vi "box detection.vi"(0 "PWM Ref In 2":T1, 1 "Angle":dbl, 2 "Distance":dbl, 3 "error in (no error) 2":errorcluster) -> (10 "error out 2":errorcluster)   [LabVIEW 2014]
uses:
  <vilib>/myRIO/Instrument Drivers/Onboard IO/PWM/typedefs/PWM Reference.ctl
  <vilib>/myRIO/Common/Instrument Driver Framework/Utilities/typedefs/myRIO Generic Hardware Reference.ctl
  <vilib>/myRIO/Common/Instrument Driver Framework/Utilities/typedefs/Hardware Version Enum.ctl
  <vilib>/myRIO/Common/Instrument Driver Framework/Utilities/typedefs/myRIO v1.0 Reference.ctl
  <vilib>/myRIO/Common/Instrument Driver Framework/Utilities/typedefs/Generic FPGA Reference.ctl
  <vilib>/myRIO/Common/Instrument Driver Framework/myRIO v1.0/PWM/typedefs/PWM Channels Enum.ctl
  <vilib>/myRIO/Instrument Drivers/Onboard IO/PWM/typedefs/PWM Configuration.ctl
  <vilib>/myRIO/Instrument Drivers/Onboard IO/AI/typedefs/AI Reference.ctl
  <vilib>/myRIO/Common/Instrument Driver Framework/myRIO v1.0/AI/typedefs/AI Channels List.ctl
  <vilib>/myRIO/Common/Instrument Driver Framework/myRIO v1.0/AI/typedefs/AI Channels Enum.ctl
  <vilib>/myRIO/Common/Instrument Driver Framework/Utilities/typedefs/Analog Scaling Constants List.ctl
  <vilib>/myRIO/Common/Instrument Driver Framework/Utilities/typedefs/Analog Scaling Constants.ctl
  <vilib>/userdefined/High Color/nirio_resource_hc.ctl
  <vilib>/myRIO/Common/Instrument Driver Framework/Utilities/vis/Is FPGA Ref Available.vi
  <vilib>/myRIO/Common/Instrument Driver Framework/myRIO v1.0/AI/vis/myRIO v1.1 Open AI.vi
  <vilib>/myRIO/Instrument Drivers/Onboard IO/AI/vis/Read.vi
  <vilib>/myRIO/Common/Instrument Driver Framework/Utilities/vis/Validate Channels.vi
  <vilib>/myRIO/Common/Instrument Driver Framework/myRIO v1.0/AI/vis/myRIO v1.0 Reserve AI.vi
  <vilib>/myRIO/Common/Instrument Driver Framework/myRIO v1.0/AI/vis/myRIO v1.0 Build MUX Configuration AI.vi
  <vilib>/myRIO/Common/Instrument Driver Framework/myRIO v1.0/Resource Manager/vis/myRIO v1.0 Reserve Channel List.vi
  <vilib>/myRIO/Common/Instrument Driver Framework/myRIO v1.0/Resource Manager/vis/myRIO v1.0 Reserve Channel.vi
  <vilib>/myRIO/Common/Instrument Driver Framework/myRIO v1.0/Resource Manager/vis/myRIO v1.0 Unreserve Channel.vi
  <vilib>/myRIO/Common/Instrument Driver Framework/myRIO v1.0/Resource Manager/vis/myRIO v1.0 Build Mutex Name.vi
  <vilib>/Utility/VariantDataType/GetNumericInfo.vi
  <vilib>/Utility/error.llb/Error Cluster From Error Code.vi
  <vilib>/myRIO/Common/Instrument Driver Framework/myRIO v1.0/myRIO v1.1 Open.vi
  <vilib>/myRIO/Common/Instrument Driver Framework/myRIO v1.0/AI/vis/myRIO v1.0 Get Scaling Constants AI.vi
  <vilib>/myRIO/Common/Instrument Driver Framework/Utilities/vis/IO Manager.vi
  <vilib>/myRIO/Common/Instrument Driver Framework/Utilities/vis/Configuration Manager.vi
  <vilib>/myRIO/Common/Instrument Driver Framework/myRIO v1.0/myRIO v1.0 Close.vi
  <vilib>/myRIO/Common/Instrument Driver Framework/myRIO v1.0/AI/vis/myRIO v1.0 Read AI.vi
  <vilib>/myRIO/Express VI/Onboard IO/AI/AI Express VI.xnode
  <vilib>/myRIO/Instrument Drivers/Onboard IO/AI/vis/myRIO AI Open.xnode
  <vilib>/ptbypt/NI_PtbyPt.lvlib
  <vilib>/myRIO/Instrument Drivers/Onboard IO/AI/AI.lvlib
  <vilib>/myRIO/Instrument Drivers/Onboard IO/PWM/PWM.lvlib
panel:
  out "color":string
  in  "Min range":dbl
  in  "Box is found":bool
  out "range":dbl format="%_3g"
  in  "Koffset [cm]":dbl
  in  "Kscale [cm-V]":dbl=27.5
  out "Vo [V]":dbl format="%.2f"
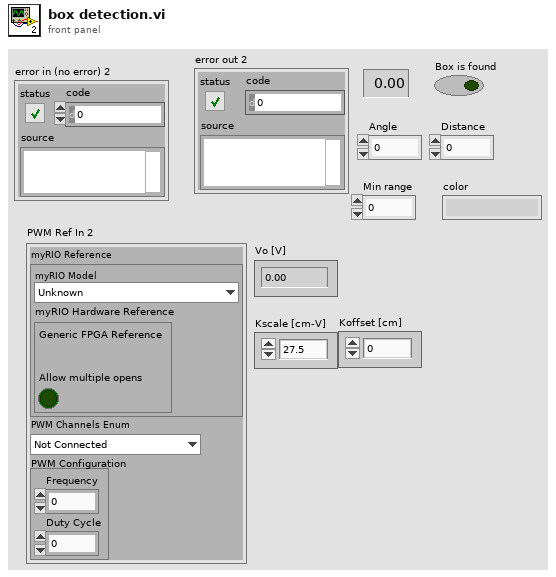
[diagram p1: front panel]
types:
  T1 = typedef "PWM.lvlib/PWM Reference.ctl" = cluster{"myRIO Reference":T2, "PWM Channels Enum":T6, "PWM Configuration":T7}
  T2 = typedef "myRIO Generic Hardware Reference.ctl" = cluster{"myRIO Model":T3, "myRIO Hardware Reference":T4}
  T3 = typedef "Hardware Version Enum.ctl" = enum16{"Unknown", "myRIO-1900", "myRIO-1950"}
  T4 = typedef "myRIO v1.0 Reference.ctl" = cluster{"Generic FPGA Reference":T5, "Allow multiple opens":bool}
  T5 = typedef "Generic FPGA Reference.ctl" = refnum<k20>
  T6 = typedef "PWM Channels Enum.ctl" = enum16{"Not Connected", "C/PWM0", "C/PWM1", "A/PWM0", "A/PWM1", "A/PWM2", "B/PWM0", "B/PWM1", "B/PWM2"}
  T7 = typedef "PWM.lvlib/PWM Configuration.ctl" = cluster{"Frequency":dbl, "Duty Cycle":dbl}
  T8 = typedef "AI.lvlib/AI Reference.ctl" = cluster{"myRIO Reference":T2, "AI Channels List":T9, "AI Scaling Constants List":T11}
  T9 = typedef "AI Channels List.ctl" = T10[]
  T10 = typedef "AI Channels Enum.ctl" = enum16{"Not Connected", "AudioIn/Left", "AudioIn/Right", "C/AI0", "C/AI1", "A/AI0", "A/AI1", "A/AI2", "A/AI3", "B/AI0", "B/AI1", "B/AI2", "B/AI3"}
  T11 = typedef "Analog Scaling Constants List.ctl" = T12[]
  T12 = typedef "Analog Scaling Constants.ctl" = cluster{"LSB Weight (Volts)":dbl, "Offset (Volts)":dbl, "Signed?":bool}
  T13 = typedef "nirio_resource_hc.ctl" = tag
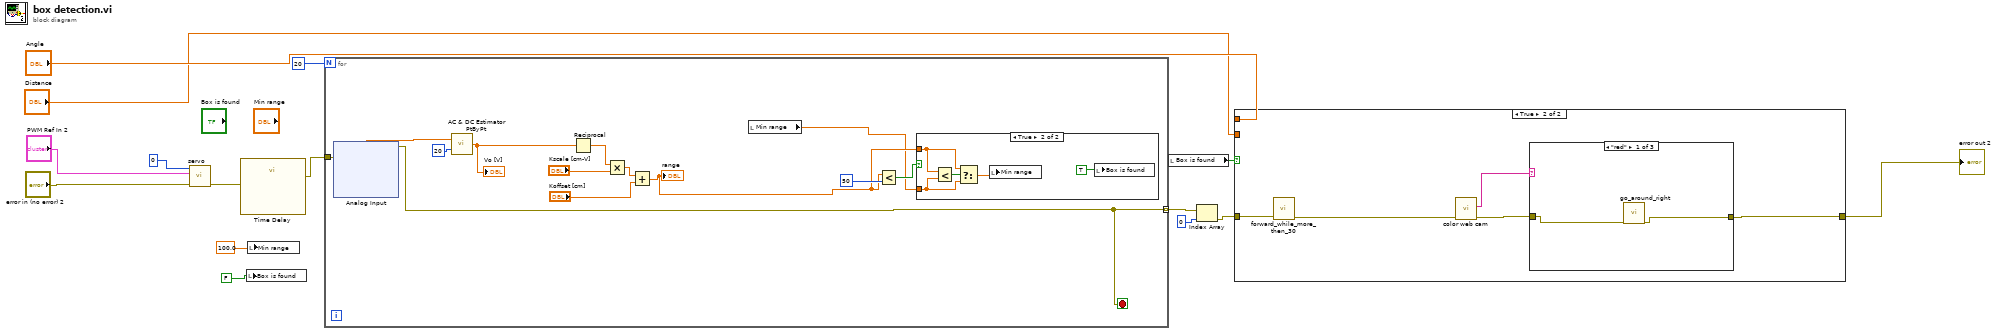
[diagram p0: block diagram]
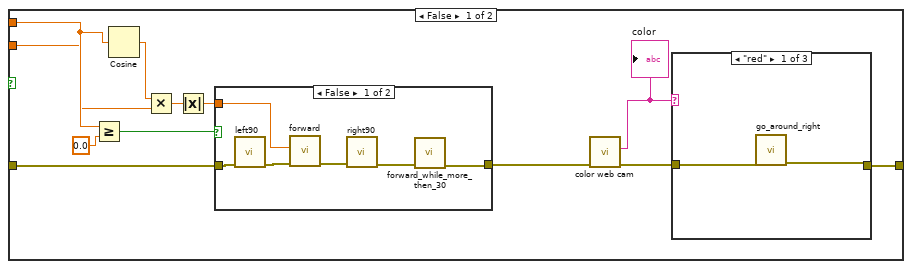
[diagram p2: hidden frame]
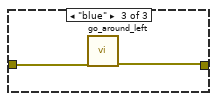
[diagram p4: hidden frame]
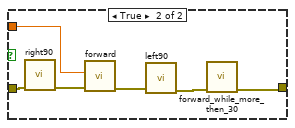
[diagram p5: hidden frame]
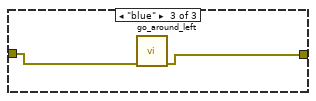
[diagram p7: hidden frame]
diagram:
  n1 = call "servo.vi"("error in (no error) 2"="error in (no error) 2", "PWM Ref In 2"="PWM Ref In 2", "Angle 2"=0) -> ("error out 2"=w12:errorcluster)  [unwired: 8 in]
  n2 = call "Time Delay"("error in (no error)"=w12) -> ("error out"=w8:errorcluster)  [unwired: 10 in]
  n3 = local write "Box is found"(FALSE) -> ()
  n4 = local write "Min range"(100.0) -> ()
  n5 = for {
    N: 20 -> [_]
    tunnel: [w18] -> w10 mode=indexing
    tunnel: w8 -> [w20]
    stop <- w18 stop-if-true
    n6 = xnode "Analog Input"("error in (no error)"=w20) -> ("A/AI0 (Pin 3)"=w25:dbl, "error out"=w18:errorcluster)
    n7 = call <vilib>:"AC & DC Estimator PtByPt.vi"("signal"=w25, "sample length"=20) -> ("DC estimate (V)"=w24:dbl)  [unwired: 1 in, 2 out]
    "Vo [V]" <- w24
    n8 = Reciprocal(x=w24) -> (1/x=w27:dbl)
    n9 = Multiply(x=w27, y="Kscale [cm-V]") -> (x*y=w21:dbl)
    n10 = Add(x=w21, y="Koffset [cm]") -> (x+y=w17:dbl)
    "range" <- w17
    n11 = local read "Min range"() -> (w16:dbl)
    n12 = Less?(x=w17, y=50) -> (x < y?=w19:bool)
    n13 = case shown="True" w19 {
      tunnel: w16 -> [_ w29]
      tunnel: w17 -> [_ w30]
      frame False {
      }
      frame True {
        n14 = Less?(x=w30, y=w29) -> (x < y?=w32:bool)
        n15 = Select(t=w30, s=w32, f=w29) -> (s? t:f=w33:dbl)
        n16 = local write "Min range"(w33) -> ()
        n17 = local write "Box is found"(TRUE) -> ()
      }
    }
  }
  n18 = local read "Box is found"() -> (w1:bool)
  n19 = Index Array(array=w10, index=0) -> (element=w6:errorcluster)
  n20 = case shown="True" w1 {
    tunnel: [w73 w102] -> w7
    tunnel: w6 -> [w82 w101]
    tunnel: "Angle" -> [w79 _]
    tunnel: "Distance" -> [w77 _]
    frame False {
      n21 = Greater Or Equal?(x=w79, y=0.0) -> (x >= y?=w81:bool)
      n22 = Cosine(x=w79) -> (cos(x)=w78:dbl)
      n23 = Multiply(x=w78, y=w77) -> (x*y=w76:dbl)
      n24 = Absolute Value(x=w76) -> (abs(x)=w71:dbl)
      n25 = case shown="False" w81 {
        tunnel: w82 -> [w93 w99]
        tunnel: [w88 w94] -> w74
        tunnel: w71 -> [w91 w97]
        frame False {
          n26 = call "left90.vi"("error in (no error)"=w93) -> ("error out"=w92:errorcluster)  [unwired: 9 in, 1 out]
          n27 = call "forward.vi"("error in (no error)"=w92, "Dist (cm)"=w91) -> ("error out"=w90:errorcluster)  [unwired: 9 in]
          n28 = call "right90.vi"("error in (no error)"=w90) -> ("error out"=w89:errorcluster)  [unwired: 10 in]
          n29 = call "forward_while_more_then_30.vi"("error in (no error)"=w89) -> ("error out"=w88:errorcluster)  [unwired: 10 in]
        }
        frame True {
          n30 = call "right90.vi"("error in (no error)"=w99) -> ("error out"=w98:errorcluster)  [unwired: 10 in]
          n31 = call "forward.vi"("error in (no error)"=w98, "Dist (cm)"=w97) -> ("error out"=w96:errorcluster)  [unwired: 9 in]
          n32 = call "left90.vi"("error in (no error)"=w96) -> ("error out"=w95:errorcluster)  [unwired: 9 in, 1 out]
          n33 = call "forward_while_more_then_30.vi"("error in (no error)"=w95) -> ("error out"=w94:errorcluster)  [unwired: 10 in]
        }
      }
      n34 = call "color web cam.vi"("error in (no error)"=w74) -> ("error out 2"=w75:errorcluster, "color"=w72:string)  [unwired: 8 in]
      "color" <- w72
      n35 = case shown="\"red\"" w72 {
        tunnel: w75 -> [w84 w85 w87]
        tunnel: [w83 w85 w86] -> w73
        frame "red" {
          n36 = call "go_around_right.vi"("error in (no error)"=w84) -> ("error out 2"=w83:errorcluster)  [unwired: 10 in]
        }
        frame Default {
        }
        frame "blue" {
          n37 = call "go_around_left.vi"("error in (no error)"=w87) -> ("error out 2"=w86:errorcluster)  [unwired: 10 in]
        }
      }
    }
    frame True {
      n38 = call "forward_while_more_then_30.vi"("error in (no error)"=w101) -> ("error out"=w100:errorcluster)  [unwired: 10 in]
      n39 = call "color web cam.vi"("error in (no error)"=w100) -> ("error out 2"=w104:errorcluster, "color"=w103:string)  [unwired: 8 in]
      n40 = case shown="\"red\"" w103 {
        tunnel: w104 -> [w106 w107 w109]
        tunnel: [w105 w107 w108] -> w102
        frame "red" {
          n41 = call "go_around_right.vi"("error in (no error)"=w106) -> ("error out 2"=w105:errorcluster)  [unwired: 10 in]
        }
        frame Default {
        }
        frame "blue" {
          n42 = call "go_around_left.vi"("error in (no error)"=w109) -> ("error out 2"=w108:errorcluster)  [unwired: 10 in]
        }
      }
    }
  }
  "error out 2" <- w7
